vi "Queue Last Ack.vi"(10 "Queue jettl":refnum<class "Queue jettl.lvclass">, 11 "Base Queue jettl in":refnum<class "Base Queue jettl.lvclass">) -> (3 "Base Queue jettl out":refnum<class "Base Queue jettl.lvclass">)   [LabVIEW 2021, in "jettl.lvlib" / "Base Queue jettl.lvlib" / "Base Queue jettl.lvclass"]
uses:
  Base Queue jettl.lvclass
  Queue jettl/Queue jettl.lvclass
  Base Queue jettl.lvclass/Base Queue jettl.ctl
  jettl.lvlib
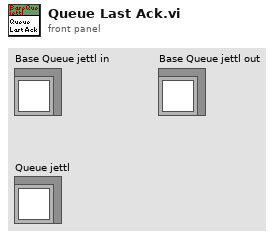
[diagram p1: front panel]
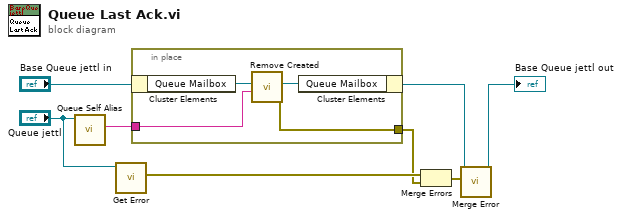
[diagram p0: block diagram]
diagram:
  n1 = call-dynamic "Queue Self Alias.vi"("jettl in"="Queue jettl") -> ("Queue Self Alias"=w2:string)  [unwired: 9 in, 1 out]
  n2 = call-dynamic "Get Error.vi"("jettl in"="Queue jettl") -> ("Error"=w8:errorcluster)  [unwired: 10 in]
  n3 = in-place {
    in-place-border: w2 -> [w10]
    in-place-border: [w9] -> w3
    n4 = in-place-cluster #1("Base Queue jettl in") -> ("Queue Mailbox"=w12:refnum<data-value>)
    n5 = call "Remove Created.vi"("Queue Self Alias"=w10, "Queue Mailbox in"=w12) -> ("error out"=w9:errorcluster, "Queue Mailbox out"=w11:refnum<data-value>)  [unwired: 8 in]
    n6 = in-place-cluster #1("Queue Mailbox"=w11) -> (w7:refnum<class "Base Queue jettl.lvclass">)
  }
  n7 = Merge Errors(w8, w3) -> (w4:errorcluster)
  n8 = call-dynamic "Merge Error.vi"("Error"=w4, "Base Queue jettl in"=w7) -> ("Base Queue jettl out"=→"Base Queue jettl out":refnum<class "Base Queue jettl.lvclass">)  [unwired: 9 in]
